vi "OFDM-SIM去除CP.vi"(1 "索引":i32, 2 "定时频偏":i32, 3 "FFT大小":i32, 4 "循环前缀大小":i32, 5 "总子载波数":i32, 6 "接收的串行数据流":cdb[](array[numeric])) -> (0 "子数组":cdb[](array[numeric]))   [LabVIEW 2018]
panel:
  out "大小":i32
  out "大小 2":i32
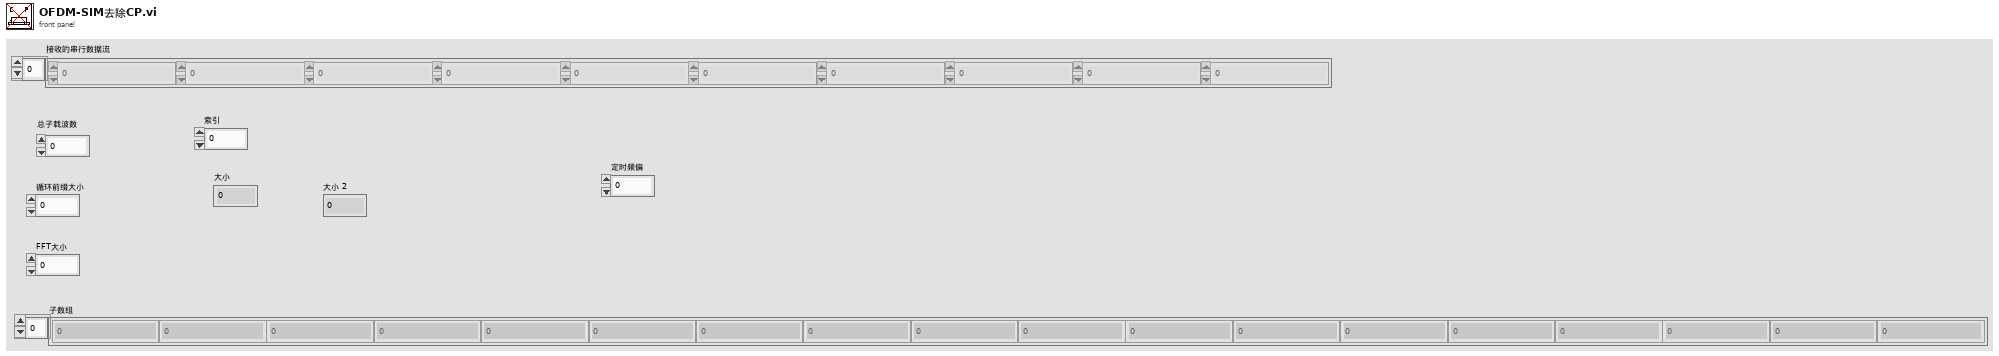
[diagram p1: front panel]
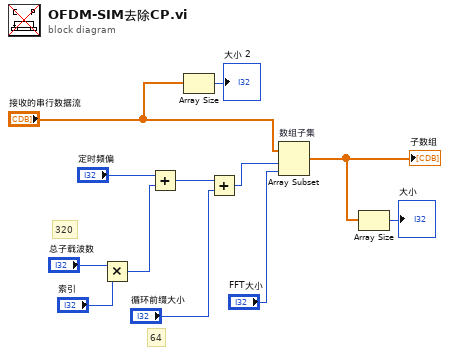
[diagram p0: block diagram]
diagram:
  # "64"
  # "320"
  n1 = Multiply(x="总子载波数", y="索引") -> (x*y=w5:i32)
  n2 = Add(x="定时频偏", y=w5) -> (x+y=w6:i32)
  n3 = Array Size(array="接收的串行数据流") -> (size(s)=→"大小 2":i32)
  n4 = Add(x=w6, y="循环前缀大小") -> (x+y=w3:i32)
  n5 = Array Subset "数组子集"(array="接收的串行数据流", index=w3, length="FFT大小") -> (w1:cdb[])
  "子数组" <- w1
  n6 = Array Size(array=w1) -> (size(s)=→"大小":i32)
